vi "Equi-Ripple BandPass.vi"   [LabVIEW 2024, in "NI_AALBase.lvlib"]
doc: "<p>Generates a bandpass FIR filter with equi-ripple characteristics using the Parks-McClellan algorithm and the <strong>higher pass freq</strong>, <strong>lower pass freq</strong>, <strong># of taps</strong>, <strong>lower stop freq</strong>, <strong>higher stop freq</strong>, and <strong>sampling freq: fs</strong>. The Equi-Ripple BandPass VI then applies a linear-phase, bandpass filter to the input sequence <strong>X</strong> using the <a href=\"nihelplauncher://docs/csh?context=lvcore_lvanls_convolution\">Convolution</a> VI to obtain <strong>Filtered X</strong>. Wire data to the <strong>X</strong> input to determine the polymorphic instance to use or <a href=\"nihelplauncher://docs/csh?context=lvcore_lvhowto_selectingdefaultinstpolyvi\">manually select</a> the instance.</p>"
uses:
  NI_AALBase.lvlib
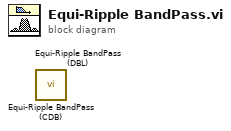
[diagram p0: block diagram]
diagram:
  n1 = call "Equi-Ripple BandPass (CDB).vi"() -> ()  [unwired: 8 in, 2 out]
  n2 = call "Equi-Ripple BandPass (DBL).vi"() -> ()  [unwired: 8 in, 2 out]
